vi "Events.vi"() -> ()   [LabVIEW 2014]
uses:
  <vilib>/Rock Robotics/WPI/Solenoid/WPI_SolenoidValue.ctl
  Eventgrab.ctl
panel:
  out "Joystick angle constant":dbl=4.2
  out "DesiredAngle":dbl
  in  "DriveMode":enum16{"Arcade", "Tank", "Mecanum"}(ring)=enum."Mecanum"
  out "Debug constants":T1
  out "Recalibrate gyro":bool
  in  "Joystick Types":T2
  out "Op Joystick":T3
  in  "Grabber":T4
  out "Shooter":T5
  out "Sensors":T7
  out "Auton Variables":cluster{"Hot?":bool, "WhichAuton":string}
  out "Shifters":cluster{"Which Gear":bool}
  out "Drive Values":T8={"Translate"=0.0, "Y-Axis (Backward Speed)"=0.0, "Rotate"=0.0, "Tank right side"=0.0, "axis 5"=0.0, "axis 6"=0.0, "Use gyro"=FALSE, "Exponential\ndrive"=TRUE, "Ring light"=FALSE, "PID rotation"=FALSE, "PID Gain"=0.0}
  # "This is where all values of robot operation are stored\nEvery device/system has it's own cluster for storing values"
  # "Don't Use Mechanium"
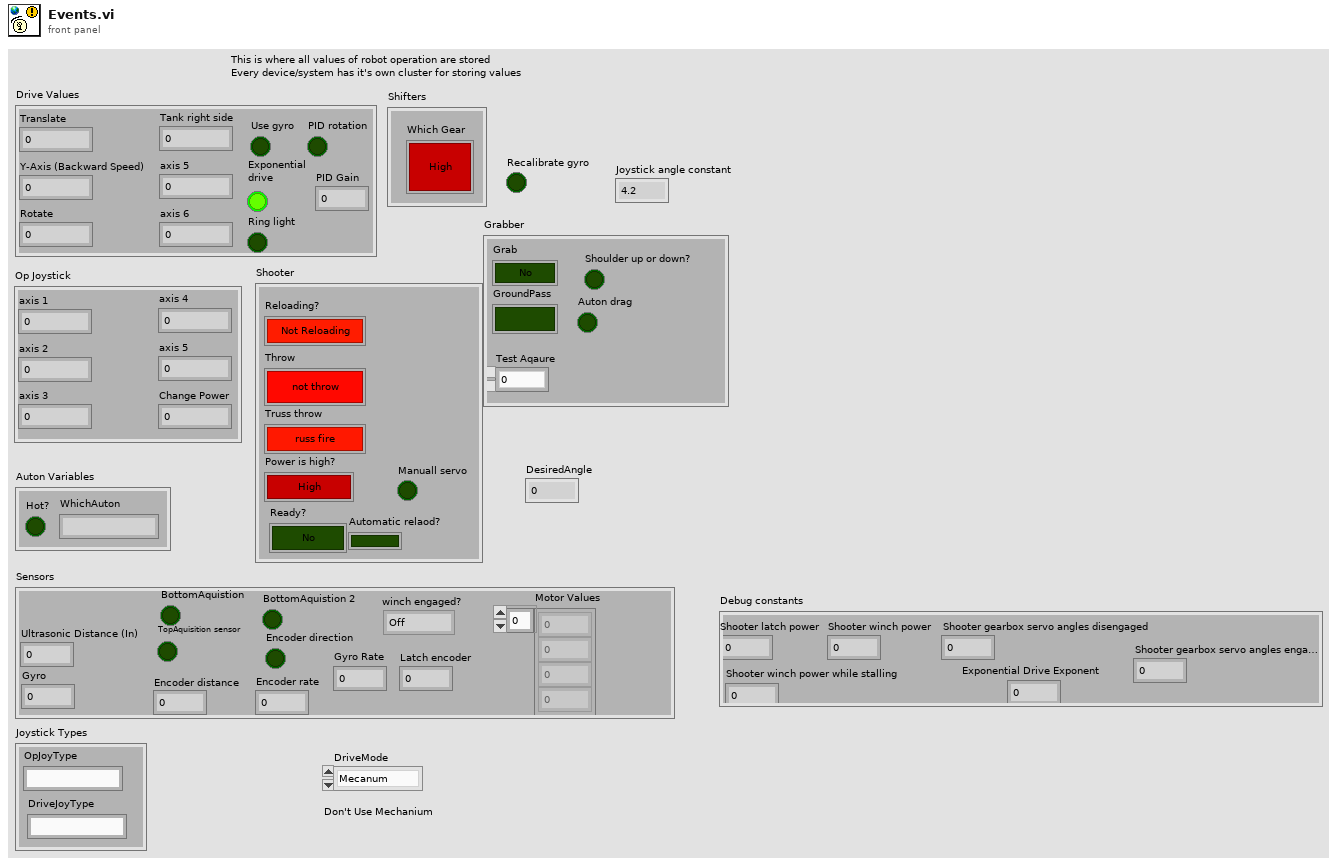
[diagram p1: front panel]
types:
  T1 = cluster{"Shooter latch power":dbl, "Shooter winch power":dbl, "Shooter gearbox servo angles disengaged":i32, "Shooter gearbox servo angles engaged":i32, "Shooter winch power while stalling":dbl, "Exponential Drive Exponent":dbl}
  T2 = cluster{"OpJoyType":string, "DriveJoyType":string}
  T3 = cluster{"axis 1":dbl, "axis 2":dbl, "axis 3":dbl, "axis 4":dbl, "axis 5":dbl, "Change Power":dbl}
  T4 = typedef "Eventgrab.ctl" = cluster{"Grab":bool, "GroundPass":bool, "Test Aqaure":dbl, "Shoulder up or down?":bool, "Auton drag":bool}
  T5 = cluster{"Reloading?":bool, "Throw":bool, "Ready?":bool, "Truss throw":bool, "Power is high?":bool, "Automatic relaod?":bool, "Manuall servo":bool}
  T6 = typedef "WPI_SolenoidValue.ctl" = enum16{"Off", "On", "Forward", "Reverse"}
  T7 = cluster{"Ultrasonic Distance (In)":dbl, "Gyro":dbl, "TopAquisition sensor":bool, "Encoder distance":dbl, "Encoder rate":dbl, "Encoder direction":bool, "winch engaged?":T6, "Motor Values":dbl[], "Latch encoder":u32, "BottomAquistion":bool, "BottomAquistion 2":bool, "Gyro Rate":dbl}
  T8 = cluster{"Translate":dbl, "Y-Axis (Backward Speed)":dbl, "Rotate":dbl, "Tank right side":dbl, "axis 5":dbl, "axis 6":dbl, "Use gyro":bool, "Exponential\ndrive":bool, "Ring light":bool, "PID rotation":bool, "PID Gain":dbl}
diagram:
